vi "FastPostParse.vi"(11 "Data":T1[](array[typedef])) -> (2 "Body":string, 3 "Status":i32)   [LabVIEW 2013, in "Advanced Plotting Toolkit.lvlib"]
uses:
  Advanced Plotting Toolkit.lvlib
  KeyValue.ctl
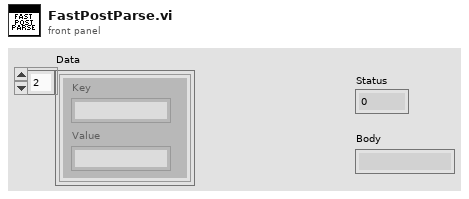
[diagram p1: front panel]
types:
  T1 = typedef "Advanced Plotting Toolkit.lvlib/KeyValue.ctl" = cluster{"Key":string, "Value":string}
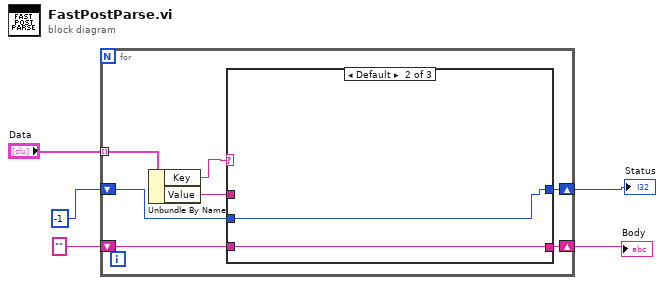
[diagram p0: block diagram]
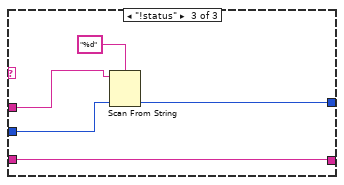
[diagram p3: hidden frame]
diagram:
  n1 = for {
    tunnel: "Data" -> [w12] mode=indexing
    shift-right: [w8] -> w2
    shift-left: -1 -> [w10]
    shift-right: [w6] -> w1
    shift-left: "" ("Body") -> [w7]
    n2 = Unbundle By Name(w12) -> ("Key"=w11:string, "Value"=w9:string)
    n3 = case shown="Default" w11 {
      tunnel: w10 -> [w14 w16 w19]
      tunnel: w9 -> [w13 _ w21]
      tunnel: [w14 w16 w18] -> w8
      tunnel: w7 -> [_ w15 w17]
      tunnel: [w13 w15 w17] -> w6
      frame "!body" {
      }
      frame Default {
      }
      frame "!status" {
        n4 = Scan From String(format string="%d", input string=w21, default 1=w19) -> (output 1=w18:i32)  [unwired: 2 in, 3 out]
      }
    }
  }
  "Status" <- w2
  "Body" <- w1
